vi "Get GUIDs from Constants VI.vi"(8 "error in":errorcluster, 11 "VI in":refnum<vi>) -> (0 "error out":errorcluster, 2 "set out":set{string}(c389), 3 "VI out":refnum<vi>)   [LabVIEW 2020, in "GUID Tool.lvlib"]
uses:
  GUID Tool.lvlib
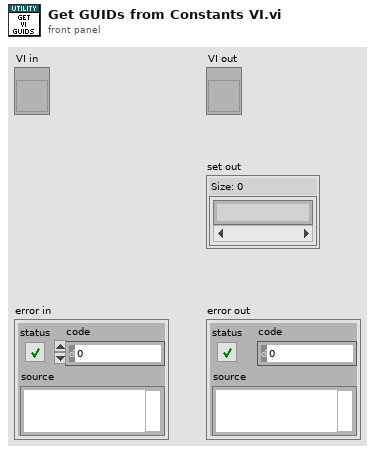
[diagram p1: front panel]
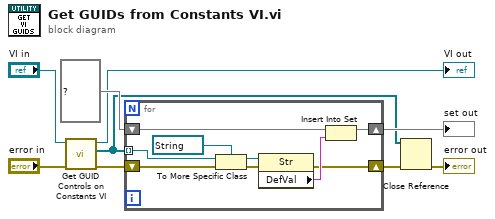
[diagram p0: block diagram]
diagram:
  n1 = call "Get GUID Controls on Constants VI.vi"("error in"="error in", "VI in"="VI in") -> ("error out"=w3:errorcluster, "GUID controls"=w1:refnum<vi>[], "VI out"=→"VI out":refnum<vi>)  [unwired: 7 in]
  n2 = for {
    tunnel: w1 -> [w18] mode=indexing
    shift-right: [w12] -> w9
    shift-left: set{string} {} ("set in") -> [w13]
    shift-right: [w11] -> w7
    shift-left: w3 -> [w10]
    n3 = To More Specific Class(target class=refnum<vi> refnum ("GUID.Import Frames"), reference=w18, error in=w10) -> (specific class reference=w16:refnum<vi>, error out=w15:errorcluster)
    n4 = property class="Str"(reference=w16, error in=w15) -> (error out=w11:errorcluster, "DefVal"=w14:string)  [unwired: 1 out]
    n5 = Insert Into Set(10:w14, 11:w13) -> (3:w12:set{string})  [unwired: 1 out]
  }
  "set out" <- w9
  n6 = Close Reference(reference=w1, error in (no error)=w7) -> (error out=→"error out":errorcluster)
